vi "TCP connect.vi"(8 "error in (no error)":errorcluster) -> (0 "error out":errorcluster, 3 "connection ID":refnum<k5>)   [LabVIEW 2019, in "ACSVcontrol-driver.lvlib"]
doc: "Initializes TCP connection and sets timeouts."
uses:
  ACSVcontrol-driver.lvlib
  Globals.vi
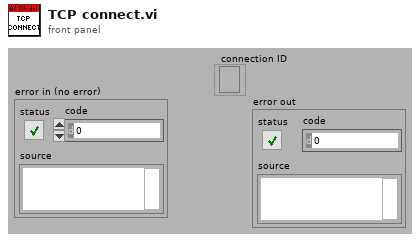
[diagram p1: front panel]
types:
  T1 = typedef "ACSVcontrol-driver.lvlib/Timeouts.ctl" = cluster{"TCP Read & Write (ms)":i32, "Sensors readout":i32, "PJVS setup":i32, "Nullmeter readout":i32, "Multiplexer setup":i32, "57XX setup":i32, "Generator setup":i32, "Synthesizer setup":i32, "Sampler readout":i32}
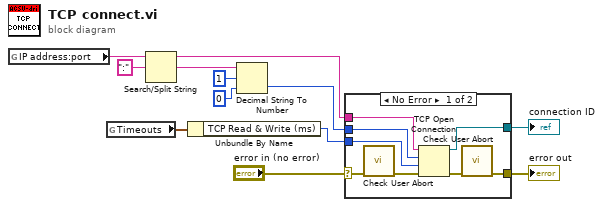
[diagram p0: block diagram]
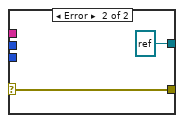
[diagram p2: hidden frame]
diagram:
  n1 = global read "Globals.vi" "IP address:port"() -> (w2:string)
  n2 = global read "Globals.vi" "Timeouts"() -> (w3:T1)
  n3 = Search/Split String(string=w2, search string/char (-)=":") -> (substring before match=w6:string, match + rest of string=w9:string)  [unwired: 1 in, 1 out]
  n4 = Unbundle By Name(w3) -> ("TCP Read & Write (ms)"=w4:i32)
  n5 = Decimal String To Number(string=w9, offset=1, default (0L)=0 ("default (0 I32)")) -> (number=w5:i32)  [unwired: 1 out]
  n6 = case shown="No Error" "error in (no error)" {
    selector: "error in (no error)" -> [w14 w21]
    tunnel: w5 -> [w20 _]
    tunnel: [w19 refnum<k5> refnum ("connection ID")] -> w12
    tunnel: w6 -> [w18 _]
    tunnel: w4 -> [w17 _]
    tunnel: [w15 w21] -> w1
    frame No Error {
      n7 = call "Check User Abort.vi"("error in (no error)"=w14) -> ("error out"=w13:errorcluster)  [unwired: 10 in]
      n8 = TCP Open Connection(address=w18, remote port or service name=w20, timeout ms (60000)=w17, error in (no error)=w13) -> (connection ID=w19:refnum<k5>, error out=w16:errorcluster)  [unwired: 1 in]
      n9 = call "Check User Abort.vi"("error in (no error)"=w16) -> ("error out"=w15:errorcluster)  [unwired: 10 in]
    }
    frame Error {
    }
  }
  "connection ID" <- w12
  "error out" <- w1
